vi "calLinFit.vi"(9 "660 Subset":dbl[](array[numeric]), 10 "532 Subset":dbl[](array[numeric]), 11 "Go3 Subset":dbl[](array[numeric])) -> (0 "cal coef":dbl format="%0.2f", 1 "660 Slope":dbl, 2 "532 slope":dbl, 3 "Calibration":cluster{dbl[], "Best Linear Fit":dbl[]}[](array[cluster]))   [LabVIEW 2011]
uses:
  <vilib>/Analysis/NI_AALPro.lvlib
  <vilib>/Analysis/NI_AALBase.lvlib
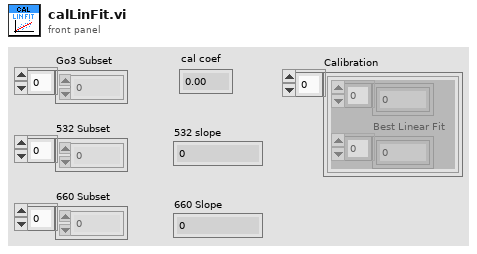
[diagram p1: front panel]
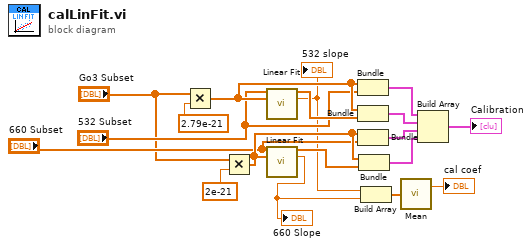
[diagram p0: block diagram]
diagram:
  n1 = Multiply(x="Go3 Subset", y=2.79e-21 ("simga-532")) -> (x*y=w10:dbl[])
  n2 = Multiply(x="Go3 Subset", y=2e-21 ("simga-532")) -> (x*y=w12:dbl[])
  n3 = call <vilib>:"Linear Fit.vi"("Y"="532 Subset", "X"=w10) -> ("Best Linear Fit"=w9:dbl[], "slope"=w4:dbl)  [unwired: 9 in, 3 out]
  "532 slope" <- w4
  n4 = call <vilib>:"Linear Fit.vi"("Y"="660 Subset", "X"=w12) -> ("Best Linear Fit"=w13:dbl[], "slope"=w3:dbl)  [unwired: 9 in, 3 out]
  "660 Slope" <- w3
  n5 = Bundle(w10, "532 Subset"="532 Subset") -> (w14:cluster{dbl[], "532 Subset":dbl[]})  [unwired: 1 in]
  n6 = Bundle(w10, "Best Linear Fit"=w9) -> (w15:cluster{dbl[], "Best Linear Fit":dbl[]})  [unwired: 1 in]
  n7 = Bundle(w12, "660 Subset"="660 Subset") -> (w16:cluster{dbl[], "660 Subset":dbl[]})  [unwired: 1 in]
  n8 = Bundle(w12, "Best Linear Fit"=w13) -> (w17:cluster{dbl[], "Best Linear Fit":dbl[]})  [unwired: 1 in]
  n9 = Build Array(w4, w3) -> (w2:dbl[])
  n10 = call <vilib>:"Mean.vi"("X"=w2) -> ("mean"=→"cal coef":dbl)  [unwired: 1 out]
  n11 = Build Array(w14, w15, w16, w17) -> (→"Calibration":cluster{dbl[], "Best Linear Fit":dbl[]}[])
